vi "Set ItemName.vi"(7 "Active Cell":cluster{"Row":i32, "Column":i32}, 8 "error in (no error)":errorcluster, 9 "ItemName":string, 10 "Popup Listbox":refnum<vi>, 11 "Multicolumn Listbox":refnum<vi>) -> (0 "error out":errorcluster)   [LabVIEW 2012]
uses:
  ListBox/Custom Type/Read and Write Mode.ctl
  Property/Set and Get Cell ItemName.vi
  Mlistbox Tools.lvlib
  ListBox/Listbox Tool.lvlib
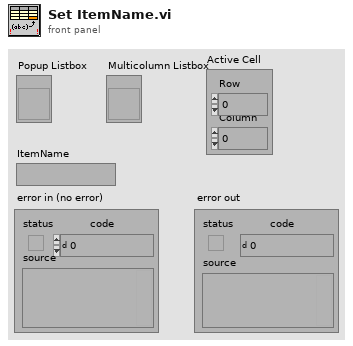
[diagram p1: front panel]
types:
  T1 = typedef "Listbox Tool.lvlib/Read and Write Mode.ctl" = enum16{"Read", "Write"}
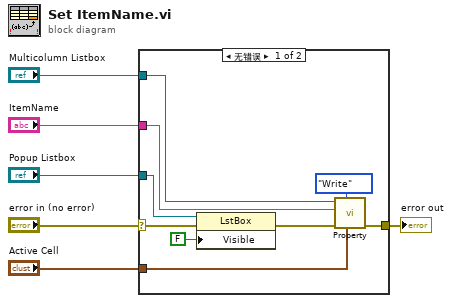
[diagram p0: block diagram]
diagram:
  n1 = case shown="无错误" "error in (no error)" {
    selector: "error in (no error)" -> [w14 w16]
    tunnel: [w13 w16] -> w5
    tunnel: "Active Cell" -> [w10 _]
    tunnel: "Multicolumn Listbox" -> [w9 _]
    tunnel: "Popup Listbox" -> [w8 _]
    tunnel: "ItemName" -> [w7 _]
    frame No Error {
      n2 = property class="LstBox"(reference=w8, error in=w14, "Visible"=FALSE) -> (error out=w11:errorcluster)  [unwired: 1 out]
      n3 = call-poly "Property.vi"("Cell"=w10, "Mode"=Read_and_Write_Mode."Write", "错误输入"=w11, "Item In"=w7, "Mlistbox Ref"=w9) -> ("错误输出"=w13:errorcluster)  [unwired: 4 in, 2 out]
    }
    frame Error {
    }
  }
  "error out" <- w5
